vi "fir1_test.vi"() -> ()   [LabVIEW 2013]
uses:
  <vilib>/rvi/FXPMathLib/FxpConvert/subVIs/nifxpmath_Convert_SimConfig.ctl
  <vilib>/fxp/LVFixedPointQuantizationPolicyTypeDef.ctl
  <vilib>/fxp/LVFixedPointOverflowPolicyTypeDef.ctl
  <vilib>/rvi/FXPMathLib/FxpConvert/simVIs/DllFxpConvertTemp_sub.vi
  <vilib>/rvi/FXPMathLib/FxpInterpret/XNode/nifxpmath_Interpret.xnode
  <vilib>/rvi/FXPMathLib/FxpConvert/XNode/nifxpmath_Convert.xnode
panel:
  out "I out":fxp<+/-,20,16>[](array[numeric])
  out "Q out":fxp<+/-,20,16>[](array[numeric])
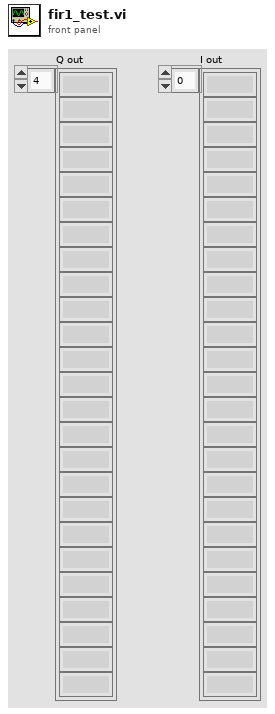
[diagram p1: front panel]
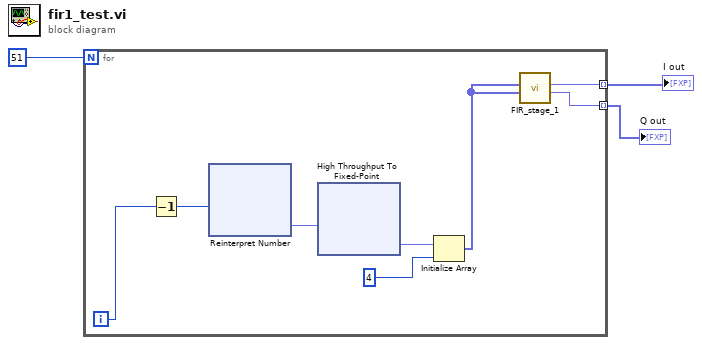
[diagram p0: block diagram]
diagram:
  n1 = for {
    N: 51 -> [_]
    tunnel: [w11] -> w3 mode=indexing
    tunnel: [w10] -> w2 mode=indexing
    i -> [w8]
    n2 = Decrement(x=w8) -> (x-1=w6:i32)
    n3 = xnode "Reinterpret Number"("x"=w6) -> ("y"=w7:fxp<+/-,32,32>)
    n4 = xnode "High Throughput To Fixed-Point"("x"=w7) -> ("y"=w5:fxp<+/-,16,14>)
    n5 = Initialize Array(w5, 4 ("dimension size")) -> (w4:fxp<+/-,16,14>[])
    n6 = call "FIR_stage_1.vi"("Q in"=w4, "I in"=w4) -> ("Q out"=w10:fxp<+/-,20,16>, "I out"=w11:fxp<+/-,20,16>)  [unwired: 8 in]
  }
  "Q out" <- w2
  "I out" <- w3
